vi "IsTimerDoneSubVI.vi"(11 "End Time (Seconds)":dbl) -> (3 "Boolean":bool)   [LabVIEW 2019]
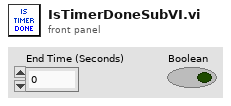
[diagram p1: front panel]
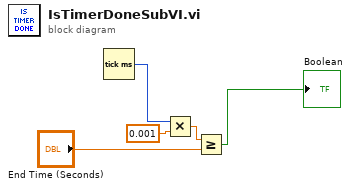
[diagram p0: block diagram]
diagram:
  n1 = Tick Count (ms)() -> (millisecond timer value=w3:u32)
  n2 = Multiply(x=w3, y=0.001) -> (x*y=w4:dbl)
  n3 = Greater Or Equal?(x=w4, y="End Time (Seconds)") -> (x >= y?=→"Boolean":bool)
